vi "Test Handle Help.vi"(11 "Instrument in":refnum<class "Instrument.lvclass">) -> (3 "Instrument out":refnum<class "Instrument.lvclass">, 8 "error out":errorcluster)   [LabVIEW 2019, in "Instrument.lvlib" / "Instrument.lvclass"]
uses:
  Instrument.lvclass
  aa6cf7f1-20d1-420b-829c-4c580da5af85.vi
panel:
  out "data":string[](array[string])
  in  "error in (no error)":errorcluster
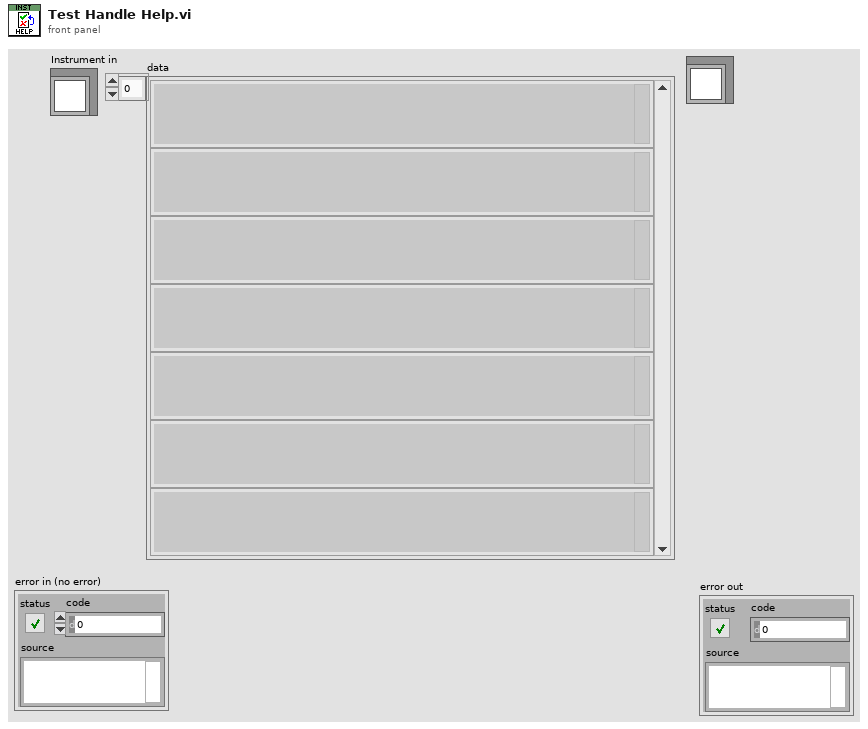
[diagram p1: front panel]
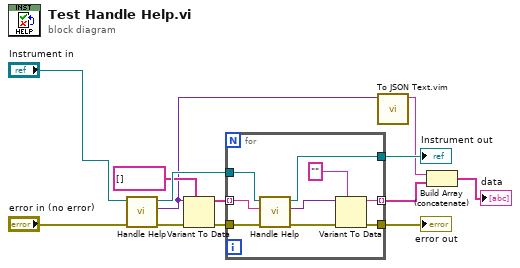
[diagram p0: block diagram]
diagram:
  n1 = call "Handle Help.vi"("error in (no error)"="error in (no error)", "Instrument in"="Instrument in") -> ("error out"=w10:errorcluster, "Help"=w3:variant, "Instrument in"=w13:refnum<class "Instrument.lvclass">)  [unwired: 7 in]
  n2 = Variant To Data(error in=w10, type=string[] [], Variant=w3) -> (data=w12:string[], error out=w9:errorcluster)
  n3 = for {
    tunnel: w13 -> [w22]
    tunnel: w12 -> [w21] mode=indexing
    tunnel: [w20] -> w11
    tunnel: w9 -> [w19]
    tunnel: [w16] -> w6
    tunnel: [w14] -> w5 mode=indexing
    n4 = call "Handle Help.vi"("error in (no error)"=w19, "Command"=w21, "Instrument in"=w22) -> ("error out"=w18:errorcluster, "Help"=w17:variant, "Instrument in"=w20:refnum<class "Instrument.lvclass">)  [unwired: 6 in]
    n5 = Variant To Data(error in=w18, type="", Variant=w17) -> (data=w14:string, error out=w16:errorcluster)
  }
  "Instrument out" <- w11
  "error out" <- w6
  n6 = call "To JSON Text.vim"("Anything"=w3) -> ("<JSON>"=w2:string)  [unwired: 9 in, 1 out]
  n7 = Build Array (concatenate)(w2, w5) -> (→"data":string[])
